vi "Test_InsertRemove.vi"(8 "error in (no error)":errorcluster, 11 "TestCase in":refnum<class "BufferedArray_Functional.lvclass">) -> (0 "error out":errorcluster, 3 "TestCase out":refnum<class "BufferedArray_Functional.lvclass">)   [LabVIEW 2009, in "BufferedArray_Functional.lvclass"]
uses:
  BufferedArray_Functional.lvclass
  source/Lists.Interfaces/String/String.lvclass
  BufferedArray_Functional.lvclass/BufferedArray_Functional.ctl
  source/Lists/List/List.lvclass
  UnitTestComparisons/UnitTestComparisons.lvlib
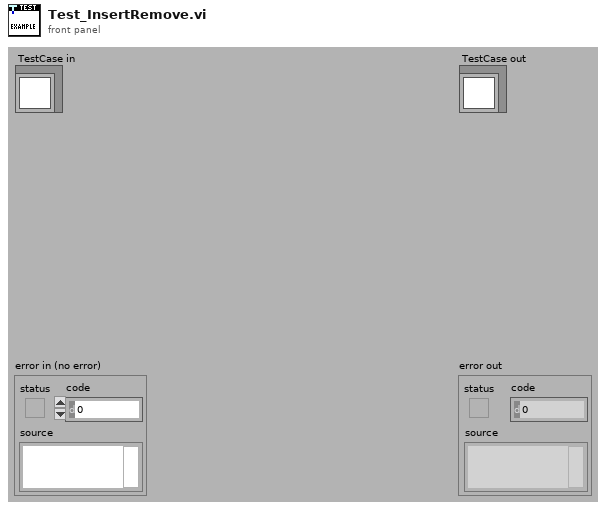
[diagram p1: front panel]
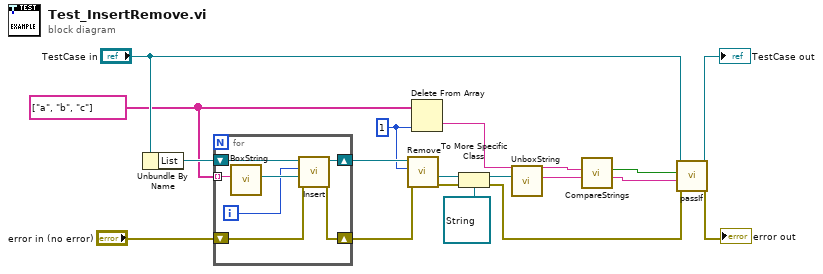
[diagram p0: block diagram]
diagram:
  w10 = 1 ("Index")
  w11 = string[] ["a", "b", "c"]
  n1 = Unbundle By Name("TestCase in") -> ("List"=w15:refnum<class "List.lvclass">)
  n2 = for {
    tunnel: w11 -> [w22] mode=indexing
    shift-right: [w24] -> w13
    shift-left: w15 -> [w25]
    shift-right: [w19] -> w12
    shift-left: "error in (no error)" -> [w20]
    i -> [w21]
    n3 = call "BoxString.vi"("String"=w22) -> ("String out"=w23:refnum<class "String.lvclass">)  [unwired: 10 in]
    n4 = call-dynamic "Insert.vi"("error in (no error)"=w20, "Item"=w23, "Index"=w21, "List in"=w25) -> ("error out"=w19:errorcluster, "List out"=w24:refnum<class "List.lvclass">)  [unwired: 6 in]
  }
  n5 = call-dynamic "Remove.vi"("error in (no error)"=w12, "Index"=w10, "List in"=w13) -> ("error out"=w8:errorcluster, "Item"=w9:refnum<class>)  [unwired: 6 in, 1 out]
  n6 = Delete From Array(array=w11, index=w10) -> (deleted portion=w4:string)  [unwired: 1 in, 1 out]
  n7 = To More Specific Class(target class=refnum<class "String.lvclass"> refnum ("LapDog.Collections.v0.Lists.Interfaces.lvlib:String.lvclass"), reference=w9, error in=w8) -> (specific class reference=w5:refnum<class "String.lvclass">, error out=w7:errorcluster)
  n8 = call "UnboxString.vi"("String in"=w5) -> ("String"=w3:string)  [unwired: 10 in]
  n9 = call "CompareStrings.vi"("Expected String"=w3, "Actual String"=w4) -> ("Message"=w1:string, "Equal?"=w2:bool)  [unwired: 8 in]
  n10 = call-dynamic "passIf.vi"("error in (no error)"=w7, "message (\"\")"=w1, "pass"=w2, "TestCase in"="TestCase in") -> ("error out"=→"error out":errorcluster, "TestCase out"=→"TestCase out":refnum<class "BufferedArray_Functional.lvclass">)  [unwired: 6 in]
